vi "Groups.Create.vi"(7 "Max Shots":T1(ring)=enum."1", 8 "error in (no error)":errorcluster, 10 "NewVal":path, 11 "Item Ref in":T2 format="%.0x") -> (0 "error out":errorcluster, 3 "Section Ref out":T2 format="%.0x")   [LabVIEW 2019, in "Fuel Injector Analysis Addon System Explorer.lvlib"]
uses:
  Fuel Injector Analysis Addon System Explorer.lvlib
  <vilib>/NI VeriStand/Custom Device API/Custom Device Item Ref.ctl
  Addon Shared/Constants.vi
  <vilib>/NI VeriStand/Custom Device API/Set Item Property (Path).vi
  <vilib>/NI VeriStand/Custom Device Tools/Custom Device Utility Library/NI VeriStand - Search for All Items by GUID.vi
  <vilib>/NI VeriStand/Custom Device API/Custom Device API.lvlib
  Addon Shared/Fuel Injector Analysis Addon Shared.lvlib
  <vilib>/NI VeriStand/Custom Device Tools/Custom Device Utility Library/Custom Device Utility Library.lvlib
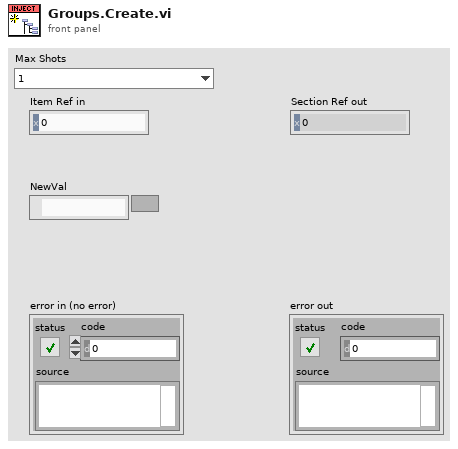
[diagram p1: front panel]
types:
  T1 = enum16{"0", "1", "2", "3", "4", "5", "6", "7", "8"}
  T2 = typedef "Custom Device API.lvlib/Custom Device Item Ref.ctl" = u64
  T3 = typedef "Fifo_DMA_Config.ctl" = cluster{"Name":string, "Depth":u32, "Write? (Deprecated:Use Implementation)":bool, "Physical Channel":u32, "Base Address":u32, "Data Width":u32, "Data Type":T4, "FXP Properties":variant, "Write Window Address":u32, "Implementation":T5, "Control Set":u32}
  T4 = typedef "niFpgaDataTypeControl.ctl" = enum32{"Boolean", "I8", "I16", "I32", "I64", "U8", "U16", "U32", "U64", "FXP", "CustomControl", "SGL"}
  T5 = typedef "niFpgaDmaChannelImplementation.ctl" = enum16{"niFpgaTargetToHost", "niFpgaHostToTarget", "niFpgaPeerToPeerWriter", "niFpgaPeerToPeerReader", "niCoreTargetToHost", "niCoreHostToTarget"}
  T6 = typedef "niFpgaBitfileStructure_VI.ctl" = cluster{"Name":string, "RegisterMap":T7[], "Icon":T12}
  T7 = typedef "nirviControlStructure.ctl" = cluster{"Name":string, "Hidden":bool, "Indicator":bool, "Flattened Type":string, "Grouping":cluster{"Grouped":bool, "Member Names":string[], "Member IDs":u32[]}, "Address":u32, "Size":u32, "Class":u32, "Internal":bool, "Typedef":T8, "ID":u32, "Bidirectional":bool, "Synchronous":bool, "Mechanical Action":T9, "Sub Controls":T10[], "Access May Timeout":bool, "Register Node":bool}
  T8 = typedef "nirviTypdefDescription.ctl" = cluster{"Typedef":bool, "Path":path}
  T9 = typedef "nirviMechanicalAction.ctl" = enum8{"Switch When Pressed", "Switch When Released", "Switch Until Released", "Latch When Pressed", "Latch When Released", "Latch Until Released"}
  T10 = typedef "nirviSubControlStructure.ctl" = cluster{"Name":string, "flattened Type":string, "Cluster Information":T11, "Typedef":T8}
  T11 = typedef "nirviClusterElementControl.ctl" = cluster{"Name Hierarchy":string[], "Item Order":u32[]}
  T12 = typedef "imagedata.ctl" = cluster{"image type":i32, "image depth":i32, "image":u8[], "mask":u8[], "colors":u32[], "Rectangle":cluster{"left":i16, "top":i16, "right":i16, "bottom":i16}}
  T13 = typedef "Fuel Injector Analysis Addon Shared.lvlib/Register.Info.ctl" = cluster{"Name":string, "Data Type":T14, "Default Value":variant}
  T14 = typedef "Fuel Injector Analysis Addon Shared.lvlib/FPGA Data Types.ctl" = enum8{"<Null>", "Injector.Core.Setting", "Injector.Global.Setting", "Injector.Mux.Setting", "Injector.Timing"}
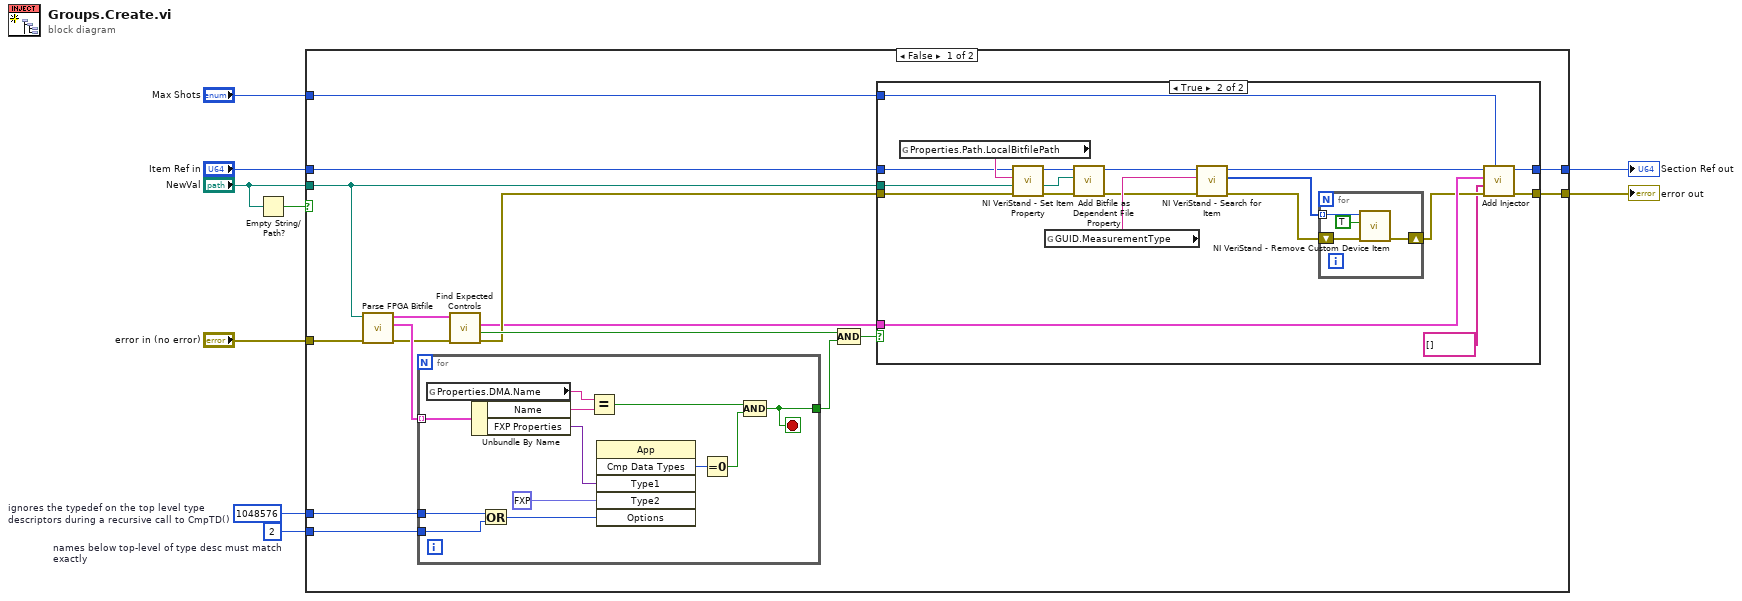
[diagram p0: block diagram]
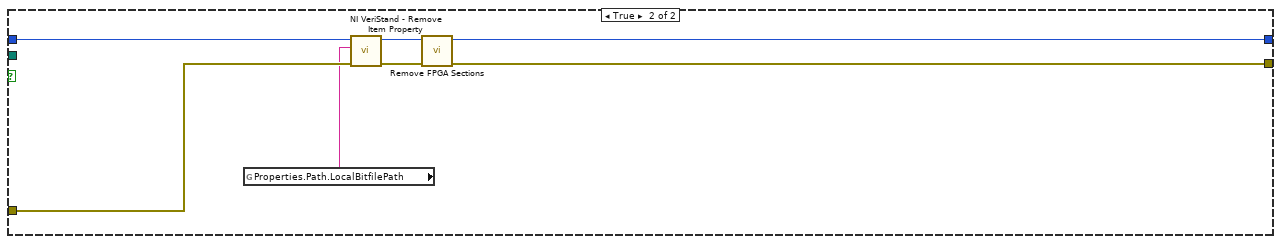
[diagram p3: hidden frame]
diagram:
  w2 = 2  # names below top-level of type desc must match exactly
  w3 = 1048576  # ignores the typedef on the top level type descriptors during a recursive call to CmpTD()
  n1 = Empty String/Path?(string/path="NewVal") -> (empty?=w7:bool)
  n2 = case shown="False" w7 {
    tunnel: "NewVal" -> [w16 _]
    tunnel: "error in (no error)" -> [w21 w67]
    tunnel: [w13 w63] -> w9
    tunnel: [w14 w62] -> w8
    tunnel: "Item Ref in" -> [w17 w68]
    tunnel: w3 -> [w23 _]
    tunnel: w2 -> [w22 _]
    tunnel: "Max Shots" -> [w10 _]
    frame False {
      n3 = call "Parse FPGA Bitfile.vi"("error in (no error)"=w21, "Path"=w16) -> ("error out"=w18:errorcluster, "DMA configuration array"=w20:T3[], "vi info"=w19:T6)  [unwired: 7 in]
      n4 = for {
        tunnel: w20 -> [w61] mode=indexing
        tunnel: [w57] -> w25
        tunnel: w23 -> [w52]
        tunnel: w22 -> [w51]
        stop <- w57 stop-if-true
        n5 = global read "Constants.vi" "Properties.DMA.Name"() -> (w59:string)
        n6 = Unbundle By Name(w61) -> ("Name"=w60:string, "FXP Properties"=w50:variant)
        n7 = Or(x=w52, y=w51) -> (x .or. y?=w56:i32)
        n8 = Equal?(x=w59, y=w60) -> (x = y?=w58:bool)
        n9 = invoke class="App" method="Cmp Data Types"("Type1"=w50, "Type2"=fxp<+/-,32,8> 0.0, "Options"=w56) -> ("Compare Data Types"=w54:i32)  [unwired: 3 in, 5 out]
        n10 = Equal To 0?(x=w54) -> (x = 0?=w53:bool)
        n11 = Compound Arithmetic op=AND(w58, w53) -> (w57:bool)
      }
      n12 = call "Find Expected Controls.vi"("error in"=w18, "vi info"=w19) -> ("error out"=w15:errorcluster, "Use?"=w24:bool, "Controls"=w11:T13[])  [unwired: 5 in, 2 out]
      n13 = Compound Arithmetic op=AND(w24, w25) -> (w12:bool)
      n14 = case shown="True" w12 {
        tunnel: w17 -> [w26 w41]
        tunnel: w16 -> [_ w44]
        tunnel: w15 -> [w27 w43]
        tunnel: [w26 w37] -> w14
        tunnel: [w27 w39] -> w13
        tunnel: w11 -> [_ w38]
        tunnel: w10 -> [_ w36]
        frame False {
        }
        frame True {
          n15 = global read "Constants.vi" "Properties.Path.LocalBitfilePath"() -> (w45:string)
          n16 = call-poly <vilib>:"NI VeriStand - Set Item Property.vi"("error in (no error)"=w43, "Value"=w44, "Property Name"=w45, "Item Ref in"=w41) -> ("error out"=w42:errorcluster, "Item Ref out"=w40:T2)  [unwired: 5 in, 1 out]
          n17 = global read "Constants.vi" "GUID.MeasurementType"() -> (w35:string)
          n18 = call "Add Bitfile as Dependent File Property.vi"("error in"=w42, "Local bitfile path"=w44, "Device Item Ref"=w40) -> ("error out"=w32:errorcluster, "Device Item Ref out"=w31:T2)  [unwired: 7 in]
          n19 = call-poly <vilib>:"NI VeriStand - Search for Item.vi"("error in"=w32, "Item GUID"=w35, "Section Ref in"=w31) -> ("error out"=w34:errorcluster, "Item Refs"=w33:T2[], "Section Ref out"=w29:T2)  [unwired: 5 in, 1 out]
          n20 = for {
            tunnel: w33 -> [w49] mode=indexing
            shift-right: [w47] -> w30
            shift-left: w34 -> [w48]
            n21 = call <vilib>:"NI VeriStand - Remove Custom Device Item.vi"("error in (no error)"=w48, "Force Delete (F)"=TRUE, "Item Ref in"=w49) -> ("error out"=w47:errorcluster)  [unwired: 7 in, 1 out]
          }
          n22 = call "Add Injector.vi"("Max Shots"=w36, "error in (no error)"=w30, "Stages"=string[] [], "Controls"=w38, "Item Ref"=w29) -> ("error out"=w39:errorcluster, "Item Ref out"=w37:T2)  [unwired: 5 in]
        }
      }
    }
    frame True {
      n23 = global read "Constants.vi" "Properties.Path.LocalBitfilePath"() -> (w66:string)
      n24 = call <vilib>:"NI VeriStand - Remove Item Property.vi"("error in (no error)"=w67, "Property Name"=w66, "Item Ref in"=w68) -> ("error out"=w64:errorcluster, "Item Ref out"=w65:T2)  [unwired: 6 in, 1 out]
      n25 = call "Remove FPGA Sections.vi"("error in (no error)"=w64, "Item Ref in"=w65) -> ("error out"=w63:errorcluster, "Item Ref out"=w62:T2)  [unwired: 8 in]
    }
  }
  "error out" <- w9
  "Section Ref out" <- w8
